vi "DPO_7K_Autoscale.vi"(7 "Thresholds":cluster{"Lower":dbl, "Upper":dbl}, 8 "Error In":errorcluster, 10 "Channel":u16(ring) items=["Channel 1", "Channel 2", "Channel 3", "Channel 4", "Math 1", "Math 2", "Math 3", "Math 4", "Reference 1", "Reference 2", "Reference 3", "Reference 4"], 11 "VISA resource name in":refnum<visa-resource-name>) -> (0 "Error Out":errorcluster, 3 "VISA resource name out":refnum<visa-resource-name>)   [LabVIEW 2020]
uses:
  DPO_7K_Autoscale_States.ctl
  subVI/Return_To_Interface.ctl
panel:
  in  "Return to Interface":T1
  # "AUTOSCALE"
  # "INPUTS"
  # "OUTPUTS"
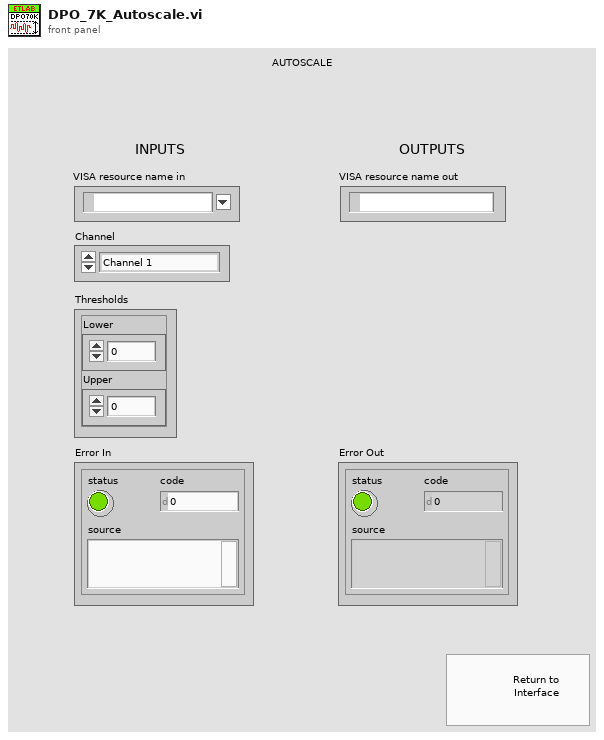
[diagram p1: front panel]
types:
  T1 = typedef "Return_To_Interface.ctl" = bool
  T2 = cluster{"Min Value":dbl, "Max Value":dbl, "Channel Scale":dbl, "Position":dbl}
  T3 = typedef "DPO_7K_Autoscale_States.ctl" = enum16{"Initial state", "Change offset", "Increase scale", "Decrease scale", "Acquisition warning", "General error", "Exit"}
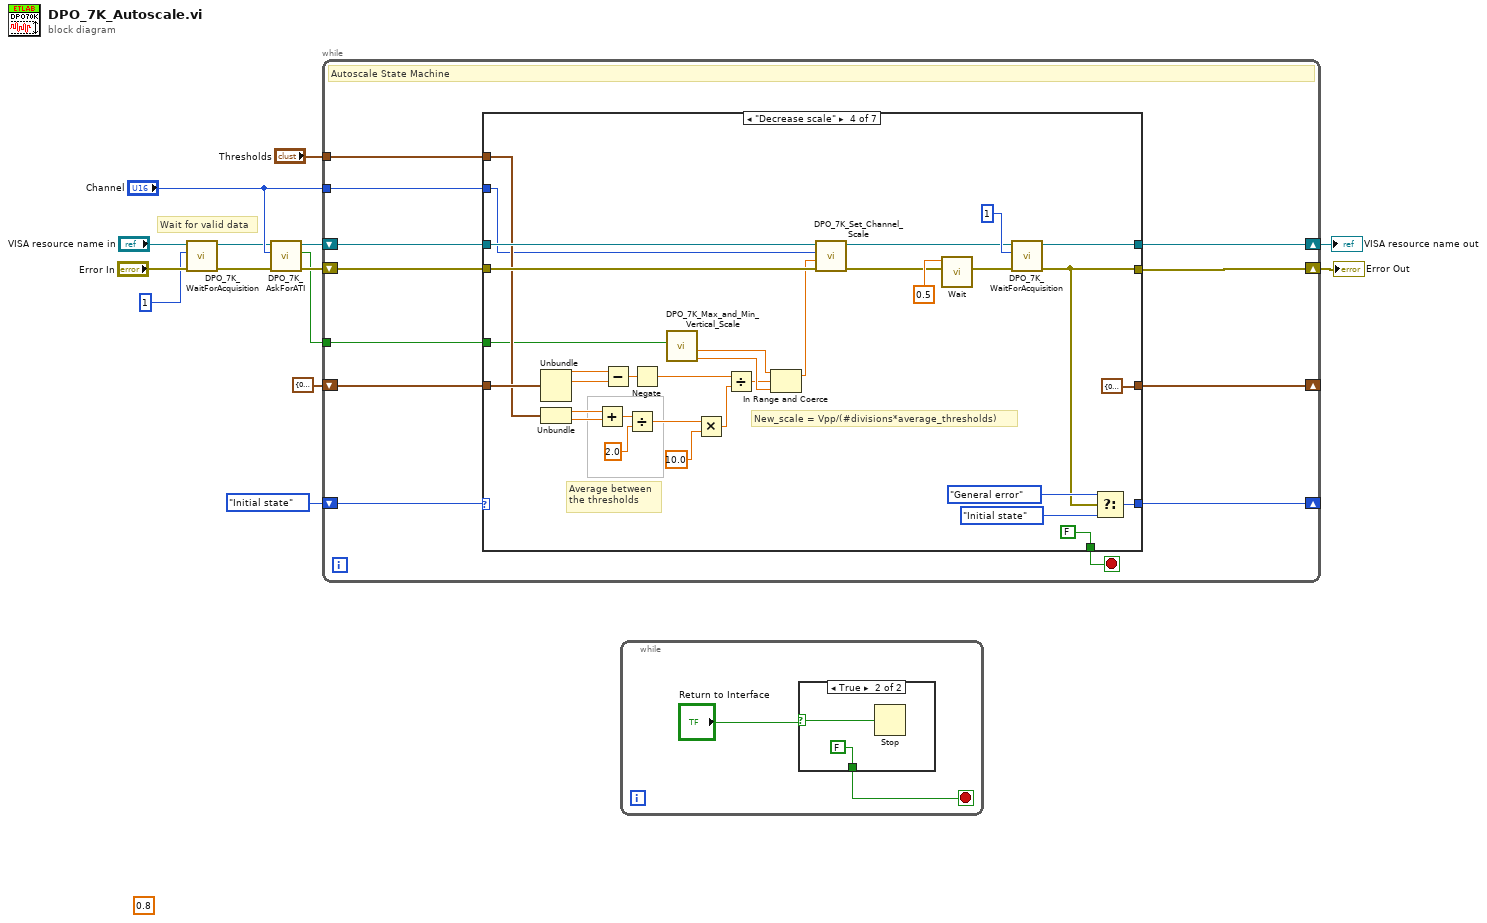
[diagram p0: block diagram]
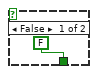
[diagram p2: hidden frame]
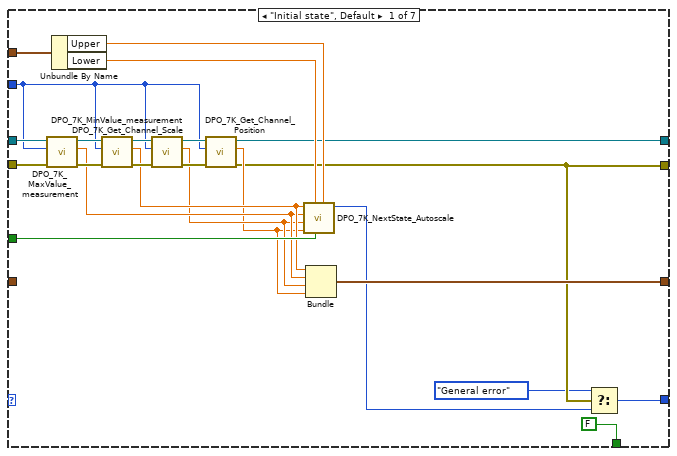
[diagram p3: hidden frame]
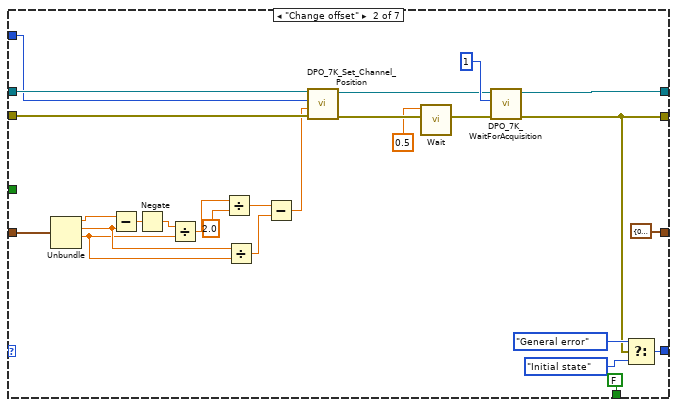
[diagram p4: hidden frame]
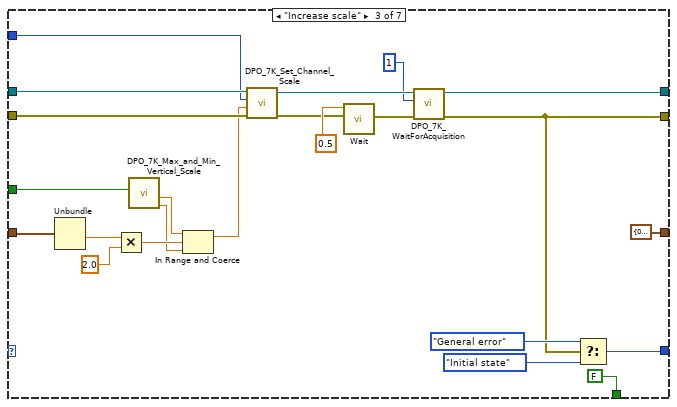
[diagram p5: hidden frame]
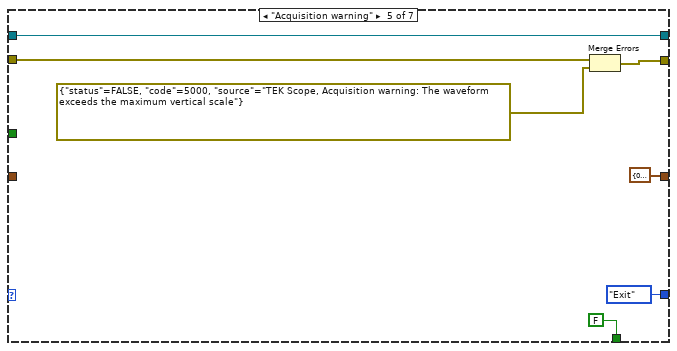
[diagram p6: hidden frame]
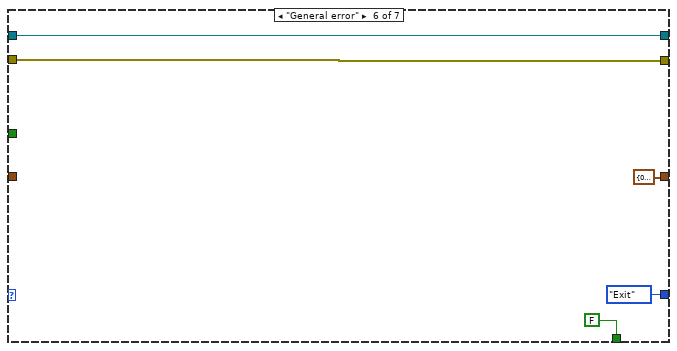
[diagram p7: hidden frame]
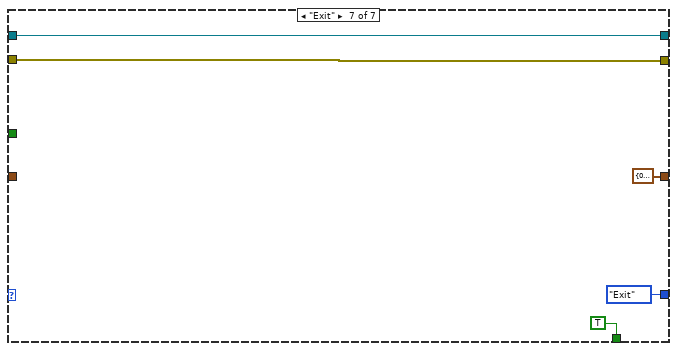
[diagram p8: hidden frame]
diagram:
  (unwired) 0.8 ("alpha")
  # "Wait for valid data"
  n1 = call "DPO_7K_WaitForAcquisition.vi"("Error In"="Error In", "Number of Waveforms"=1, "VISA resource name in"="VISA resource name in") -> ("Error Out"=w4:errorcluster, "VISA resource name out"=w5:refnum<visa-resource-name>)  [unwired: 7 in]
  n2 = call "DPO_7K_AskForATI.vi"("Error In"=w4, "Channel"="Channel", "VISA resource name in"=w5) -> ("Error Out"=w11:errorcluster, "ATI?"=w10:bool, "VISA resource name out"=w12:refnum<visa-resource-name>)  [unwired: 6 in]
  n3 = while {
    shift-right: [w25] -> w6
    shift-left: w11 -> [w26]
    shift-right: [w24] -> w7
    shift-left: w12 -> [w23]
    tunnel: "Thresholds" -> [w22]
    shift-right: [w19] -> _
    shift-left: DPO_7K_Autoscale_States."Initial state" ("Autoscale States") -> [w21]
    tunnel: w10 -> [w20]
    tunnel: "Channel" -> [w18]
    shift-right: [w16] -> _
    shift-left: T2 {"Min Value"=0.0, "Max Value"=0.0, "Channel Scale"=0.0, "Position"=0.0} -> [w15]
    stop <- w17 stop-if-true
    # "Autoscale State Machine"
    n4 = case shown="\"Decrease scale\"" w21 {
      tunnel: w26 -> [w50 w71 w98 w131 w138 w143 w145]
      tunnel: [w30 w51 w80 w101 w137 w143 w145] -> w25
      tunnel: [w36 w52 w78 w100 w139 w144 w146] -> w24
      tunnel: w23 -> [w49 w72 w99 w132 w139 w144 w146]
      tunnel: w22 -> [w48 _ _ w126 _ _ _]
      tunnel: w20 -> [w41 _ w93 w114 _ _ _]
      tunnel: [w27 w65 w86 w110 DPO_7K_Autoscale_States."Exit" ("Autoscale States") DPO_7K_Autoscale_States."Exit" ("Autoscale States") DPO_7K_Autoscale_States."Exit" ("Autoscale States")] -> w19
      tunnel: w18 -> [w38 w59 w89 w108 _ _ _]
      tunnel: [FALSE FALSE FALSE FALSE FALSE FALSE TRUE] -> w17
      tunnel: [w31 T2 {"Min Value"=0.0, "Max Value"=0.0, "Channel Scale"=0.0, "Position"=0.0} T2 {"Min Value"=0.0, "Max Value"=0.0, "Channel Scale"=0.0, "Position"=0.0} T2 {"Min Value"=0.0, "Max Value"=0.0, "Channel Scale"=0.0, "Position"=0.0} T2 {"Min Value"=0.0, "Max Value"=0.0, "Channel Scale"=0.0, "Position"=0.0} T2 {"Min Value"=0.0, "Max Value"=0.0, "Channel Scale"=0.0, "Position"=0.0} T2 {"Min Value"=0.0, "Max Value"=0.0, "Channel Scale"=0.0, "Position"=0.0}] -> w16
      tunnel: w15 -> [_ w70 w97 w130 _ _ _]
      frame "Initial state", Default {
        n5 = call "DPO_7K_MaxValue_measurement.vi"("Error In"=w50, "Channel"=w38, "VISA resource name in"=w49) -> ("Error Out"=w47:errorcluster, "Max Value"=w34:dbl, "VISA resource name out"=w46:refnum<visa-resource-name>)  [unwired: 6 in]
        n6 = Unbundle By Name(w48) -> ("Upper"=w43:dbl, "Lower"=w42:dbl)
        n7 = call "DPO_7K_MinValue_measurement.vi"("Error In"=w47, "Channel"=w38, "VISA resource name in"=w46) -> ("Error Out"=w44:errorcluster, "Min Value"=w35:dbl, "VISA resource name out"=w45:refnum<visa-resource-name>)  [unwired: 6 in]
        n8 = call "DPO_7K_Get_Channel_Scale.vi"("Error In"=w44, "Channel"=w38, "VISA resource name in"=w45) -> ("Error Out"=w39:errorcluster, "Channel Scale"=w33:dbl, "VISA resource name out"=w40:refnum<visa-resource-name>)  [unwired: 6 in]
        n9 = call "DPO_7K_Get_Channel_Position.vi"("Error In"=w39, "Channel"=w38, "VISA resource name in"=w40) -> ("Error Out"=w30:errorcluster, "Position"=w32:dbl, "VISA resource name out"=w36:refnum<visa-resource-name>)  [unwired: 6 in]
        n10 = call "DPO_7K_NextState_Autoscale.vi"("Upper Threshold"=w43, "ATI?"=w41, "Lower Threshold"=w42, "Offset"=w32, "Current Vertical Scale"=w33, "Waveform Maximum Value"=w34, "Waveform Minumum Value"=w35) -> ("Autoscale States"=w29:T3)  [unwired: 4 in]
        n11 = Bundle("Min Value"=w35, "Max Value"=w34, "Channel Scale"=w33, "Position"=w32) -> (w31:T2)  [unwired: 1 in]
        n12 = Select(t=DPO_7K_Autoscale_States."General error", s=w30, f=w29) -> (s? t:f=w27:T3)
      }
      frame "Change offset" {
        n13 = Unbundle(w70) -> ("Min Value"=w69:dbl, "Max Value"=w66:dbl, "Channel Scale"=w60:dbl)  [unwired: 1 out]
        n14 = Subtract(x=w69, y=w66) -> (x-y=w68:dbl)
        n15 = Negate(x=w68) -> (-x=w67:dbl)
        n16 = Divide(x=w67, y=w60) -> (x/y=w76:dbl)
        n17 = Divide(x=w76, y=2.0) -> (x/y=w74:dbl)
        n18 = Divide(x=w66, y=w60) -> (x/y=w73:dbl)
        n19 = Subtract(x=w74, y=w73) -> (x-y=w58:dbl)
        n20 = call "DPO_7K_Set_Channel_Position.vi"("Error In"=w71, "Position"=w58, "Channel"=w59, "VISA resource name in"=w72) -> ("Error Out"=w54:errorcluster, "VISA resource name out"=w55:refnum<visa-resource-name>)  [unwired: 6 in]
        n21 = call "Wait.vi"("Error In"=w54, "Seconds"=0.5) -> ("Error Out"=w57:errorcluster)  [unwired: 9 in]
        n22 = call "DPO_7K_WaitForAcquisition.vi"("Error In"=w57, "Number of Waveforms"=1, "VISA resource name in"=w55) -> ("Error Out"=w51:errorcluster, "VISA resource name out"=w52:refnum<visa-resource-name>)  [unwired: 7 in]
        n23 = Select(t=DPO_7K_Autoscale_States."General error" ("Autoscale States"), s=w51, f=DPO_7K_Autoscale_States."Initial state" ("Autoscale States")) -> (s? t:f=w65:T3)
      }
      frame "Increase scale" {
        n24 = Unbundle(w97) -> ("Channel Scale"=w96:dbl)  [unwired: 3 out]
        n25 = Multiply(x=w96, y=2.0) -> (x*y=w94:dbl)
        n26 = call "DPO_7K_Max_and_Min_Vertical_Scale.vi"("ATI?"=w93) -> ("Min"=w91:dbl, "Max"=w92:dbl)  [unwired: 9 in]
        n27 = In Range and Coerce(upper limit=w92, x=w94, lower limit=w91) -> (coerced(x)=w90:dbl)  [unwired: 1 out]
        n28 = call "DPO_7K_Set_Channel_Scale.vi"("Error In"=w98, "Channel Scale"=w90, "Channel"=w89, "VISA resource name in"=w99) -> ("Error Out"=w82:errorcluster, "VISA resource name out"=w79:refnum<visa-resource-name>)  [unwired: 6 in]
        n29 = call "Wait.vi"("Error In"=w82, "Seconds"=0.5) -> ("Error Out"=w81:errorcluster)  [unwired: 9 in]
        n30 = call "DPO_7K_WaitForAcquisition.vi"("Error In"=w81, "Number of Waveforms"=1, "VISA resource name in"=w79) -> ("Error Out"=w80:errorcluster, "VISA resource name out"=w78:refnum<visa-resource-name>)  [unwired: 7 in]
        n31 = Select(t=DPO_7K_Autoscale_States."General error" ("Autoscale States"), s=w80, f=DPO_7K_Autoscale_States."Initial state" ("Autoscale States")) -> (s? t:f=w86:T3)
      }
      frame "Decrease scale" {
        # "New_scale = Vpp/(#divisions*average_thresholds)"
        # "Average between\nthe thresholds"
        n32 = Unbundle(w130) -> ("Min Value"=w128:dbl, "Max Value"=w129:dbl)  [unwired: 2 out]
        n33 = Unbundle(w126) -> ("Lower"=w125:dbl, "Upper"=w124:dbl)
        n34 = Add(x=w125, y=w124) -> (x+y=w123:dbl)
        n35 = Subtract(x=w128, y=w129) -> (x-y=w127:dbl)
        n36 = Divide(x=w123, y=2.0) -> (x/y=w121:dbl)
        n37 = Negate(x=w127) -> (-x=w119:dbl)
        n38 = call "DPO_7K_Max_and_Min_Vertical_Scale.vi"("ATI?"=w114) -> ("Min"=w116:dbl, "Max"=w117:dbl)  [unwired: 9 in]
        n39 = Multiply(x=w121, y=10.0) -> (x*y=w118:dbl)
        n40 = Divide(x=w119, y=w118) -> (x/y=w115:dbl)
        n41 = In Range and Coerce(upper limit=w117, x=w115, lower limit=w116) -> (coerced(x)=w107:dbl)  [unwired: 1 out]
        n42 = call "DPO_7K_Set_Channel_Scale.vi"("Error In"=w131, "Channel Scale"=w107, "Channel"=w108, "VISA resource name in"=w132) -> ("Error Out"=w102:errorcluster, "VISA resource name out"=w103:refnum<visa-resource-name>)  [unwired: 6 in]
        n43 = call "Wait.vi"("Error In"=w102, "Seconds"=0.5) -> ("Error Out"=w106:errorcluster)  [unwired: 9 in]
        n44 = call "DPO_7K_WaitForAcquisition.vi"("Error In"=w106, "Number of Waveforms"=1, "VISA resource name in"=w103) -> ("Error Out"=w101:errorcluster, "VISA resource name out"=w100:refnum<visa-resource-name>)  [unwired: 7 in]
        n45 = Select(t=DPO_7K_Autoscale_States."General error" ("Autoscale States"), s=w101, f=DPO_7K_Autoscale_States."Initial state" ("Autoscale States")) -> (s? t:f=w110:T3)
      }
      frame "Acquisition warning" {
        n46 = Merge Errors(w138, errorcluster {"status"=FALSE, "code"=5000, "source"="TEK Scope, Acquisition warning: The waveform exceeds the maximum vertical scale"} ("error constant")) -> (w137:errorcluster)
      }
      frame "General error" {
      }
      frame "Exit" {
      }
    }
  }
  "VISA resource name out" <- w7
  "Error Out" <- w6
  n47 = while {
    stop <- w150 stop-if-true
    n48 = case shown="True" "Return to Interface" {
      selector: "Return to Interface" -> [_ w153]
      tunnel: [FALSE FALSE] -> w150
      frame False {
      }
      frame True {
        n49 = Stop(stop? (T)=w153) -> ()
      }
    }
  }
